vi "Lab08MainVI.vi"() -> ()   [LabVIEW 2022 SP3]
uses:
  VendingMachineControl.ctl
panel:
  out "Cost of a soda":dbl=0.75
  out "Enough $?":bool
  in  "$0.05":bool
  in  "$0.10":bool
  in  "Return":bool
  in  "Coke":bool
  in  "Pepsi":bool
  in  "stop":bool
  out "UI Indicator":string
  out "Current State":T1
  out "Value Deposited":dbl
  out "Change Returned":dbl
  in  "$0.25":bool
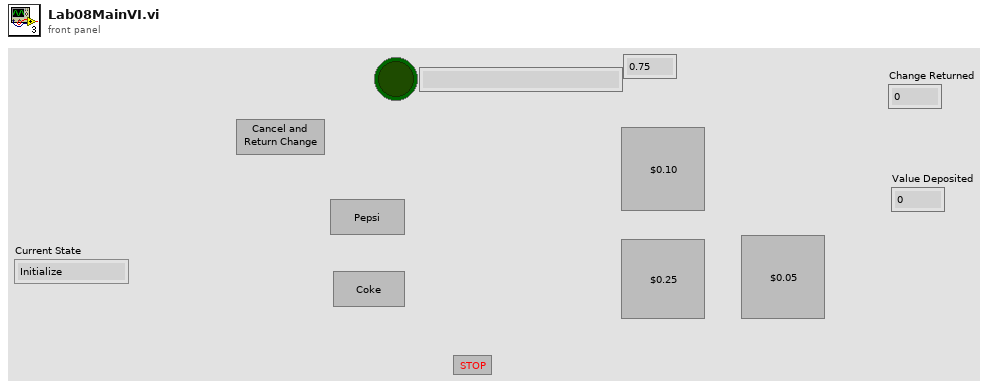
[diagram p1: front panel]
types:
  T1 = typedef "VendingMachineControl.ctl" = enum16{"Initialize", "Stop", "Wait for UI", "Deposit Soda", "Return"}
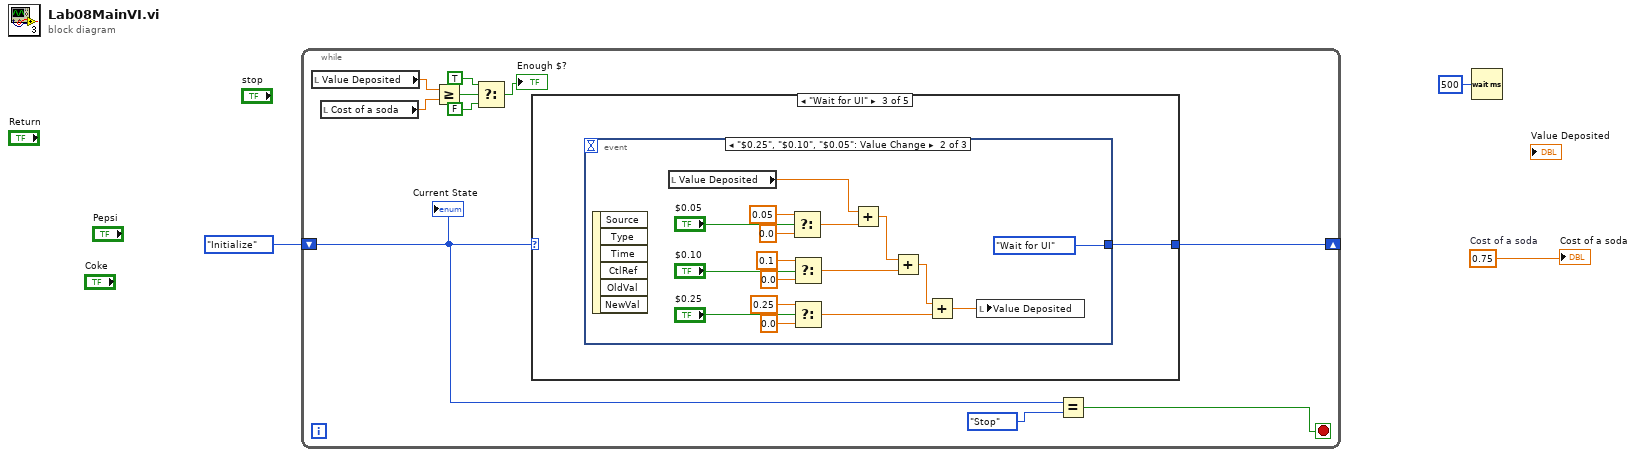
[diagram p0: block diagram]
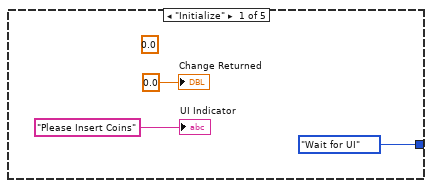
[diagram p2: hidden frame]
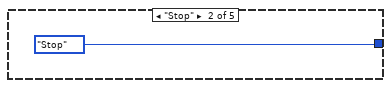
[diagram p3: hidden frame]
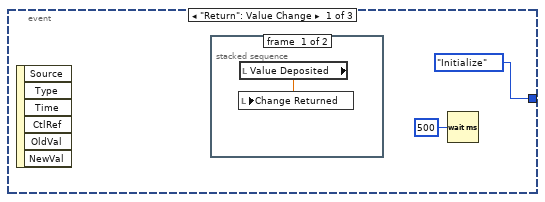
[diagram p4: hidden frame]
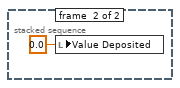
[diagram p5: hidden frame]
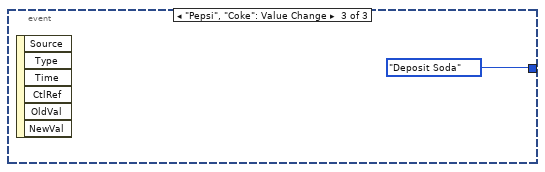
[diagram p6: hidden frame]
diagram:
  w1 = 0.75  # Cost of a soda
  n1 = while {
    shift-right: [w13] -> _
    shift-left: VendingMachineControl."Initialize" -> [w5]
    stop <- w4 stop-if-true
    n2 = local read "Value Deposited"() -> (w12:dbl)
    n3 = local read "Cost of a soda"() -> (w11:dbl)
    n4 = Greater Or Equal?(x=w12, y=w11) -> (x >= y?=w10:bool)
    n5 = Select(t=TRUE, s=w10, f=FALSE) -> (s? t:f=→"Enough $?":bool)
    n6 = case shown="\"Wait for UI\"" w5 {
      tunnel: [VendingMachineControl."Wait for UI" VendingMachineControl."Stop" w18 _ _] -> w13
      frame "Initialize" {
        (unwired) 0.0 ("Numeric 2")
        "Change Returned" <- 0.0 ("Numeric")
        "UI Indicator" <- "Please Insert Coins" ("String")
      }
      frame "Stop" {
      }
      frame "Wait for UI" {
        n7 = event shown="[1] \"$0.25\", \"$0.10\", \"$0.05\": Value Change" {
          selector: _ -> [_ _ _]
          dyn-events: _ -> [_ _ _]
          timeout: _ -> [_ _ _]
          tunnel: [VendingMachineControl."Initialize" VendingMachineControl."Wait for UI" VendingMachineControl."Deposit Soda"] -> w18
          event "Return": Value Change {
            n8 = event-data() -> ()  [unwired: 1 in, 6 out]
            n9 = stacked-sequence {
              frame #0 {
                n10 = local read "Value Deposited"() -> (w21:dbl)
                n11 = local write "Change Returned"(w21) -> ()
              }
              frame #1 {
                n12 = local write "Value Deposited"(0.0 ("Value Deposited")) -> ()
              }
            }
            n13 = Wait (ms)(milliseconds to wait=u32 500) -> ()  [unwired: 1 out]
          }
          event "$0.25", "$0.10", "$0.05": Value Change {
            n14 = event-data() -> ()  [unwired: 1 in, 6 out]
            n15 = local read "Value Deposited"() -> (w29:dbl)
            n16 = Select(t=0.05, s="$0.05", f=0.0) -> (s? t:f=w28:dbl)
            n17 = Select(t=0.1, s="$0.10", f=0.0) -> (s? t:f=w27:dbl)
            n18 = Select(t=0.25, s="$0.25", f=0.0) -> (s? t:f=w26:dbl)
            n19 = Add(x=w29, y=w28) -> (x+y=w25:dbl)
            n20 = Add(x=w25, y=w27) -> (x+y=w24:dbl)
            n21 = Add(x=w24, y=w26) -> (x+y=w23:dbl)
            n22 = local write "Value Deposited"(w23) -> ()
          }
          event "Pepsi", "Coke": Value Change {
            n23 = event-data() -> ()  [unwired: 1 in, 6 out]
          }
        }
      }
      frame "Deposit Soda" {
      }
      frame "Return" {
      }
    }
    n24 = Equal?(x=w5, y=VendingMachineControl."Stop") -> (x = y?=w4:bool)
    "Current State" <- w5
  }
  n25 = Wait (ms)(milliseconds to wait=u32 500) -> ()  [unwired: 1 out]
  "Cost of a soda" <- w1
